vi "svl_Limit Testing (array).vi"(9 "lower limit":dbl[](array[numeric]) format="%.2f", 10 "input array":dbl[](array[numeric]) format="%.2f", 11 "upper limit":dbl[](array[numeric]) format="%.2f") -> (1 "dup lower limit":dbl[](array[numeric]) format="%.2f", 2 "failure array":dbl[](array[numeric]) format="%.2f", 3 "dup upper limit":dbl[](array[numeric]) format="%.2f", 4 "test passed":bool, 6 "test results":bool[](array[boolean]))   [LabVIEW 2017, in "SoundVib_LimitTest.lvlib"]
uses:
  <vilib>/addons/Sound and Vibration/svt_Limit Test/SoundVib_LimitTest.lvlib
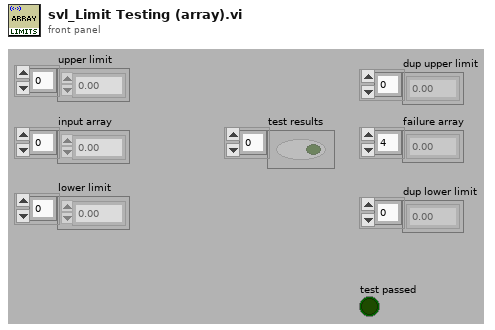
[diagram p1: front panel]
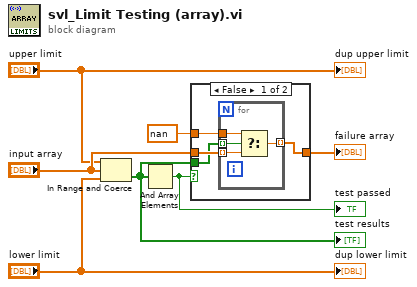
[diagram p0: block diagram]
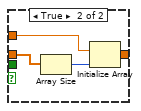
[diagram p2: hidden frame]
diagram:
  n1 = In Range and Coerce(upper limit="upper limit", x="input array", lower limit="lower limit") -> (In Range?=w7:bool[])  [unwired: 1 out]
  "test results" <- w7
  n2 = And Array Elements(Boolean array=w7) -> (logical AND=w4:bool)
  "test passed" <- w4
  n3 = case shown="False" w4 {
    tunnel: w7 -> [w10 _]
    tunnel: "input array" -> [w11 w16]
    tunnel: [w9 w17] -> w6
    tunnel: nan ("element") -> [w8 w18]
    frame False {
      n4 = for {
        tunnel: w11 -> [w13] mode=indexing
        tunnel: w10 -> [w15] mode=indexing
        tunnel: w8 -> [w12]
        tunnel: [w14] -> w9 mode=indexing
        n5 = Select(t=w12, s=w15, f=w13) -> (s? t:f=w14:dbl)
      }
    }
    frame True {
      n6 = Array Size(array=w16) -> (size(s)=w19:i32)
      n7 = Initialize Array(w18, w19) -> (w17:dbl[])
    }
  }
  "failure array" <- w6
  "dup upper limit" <- "upper limit"
  "dup lower limit" <- "lower limit"
